vi "布线趋势图示-单根.vi"(0 "基本信息":T2, 1 "布线前甩线":string[][](table), 2 "布线点位":string[][](table), 3 "布线后甩线":string[][](table), 4 "轨迹选择":u16(ring) items=["显示单根轨迹", "显示全部轨迹"]) -> (14 "引用句柄输出":T1)   [LabVIEW 2014]
uses:
  <vilib>/vision/Image Controls.llb/IMAQ Image.ctl
panel:
  out "x-y 2":dbl
  out "x-y":dbl
  out "YMIN":dbl
  out "XMIN":dbl
  out "YMAX":dbl
  out "XMAX":dbl
  out "Image":T1(plugin-control)
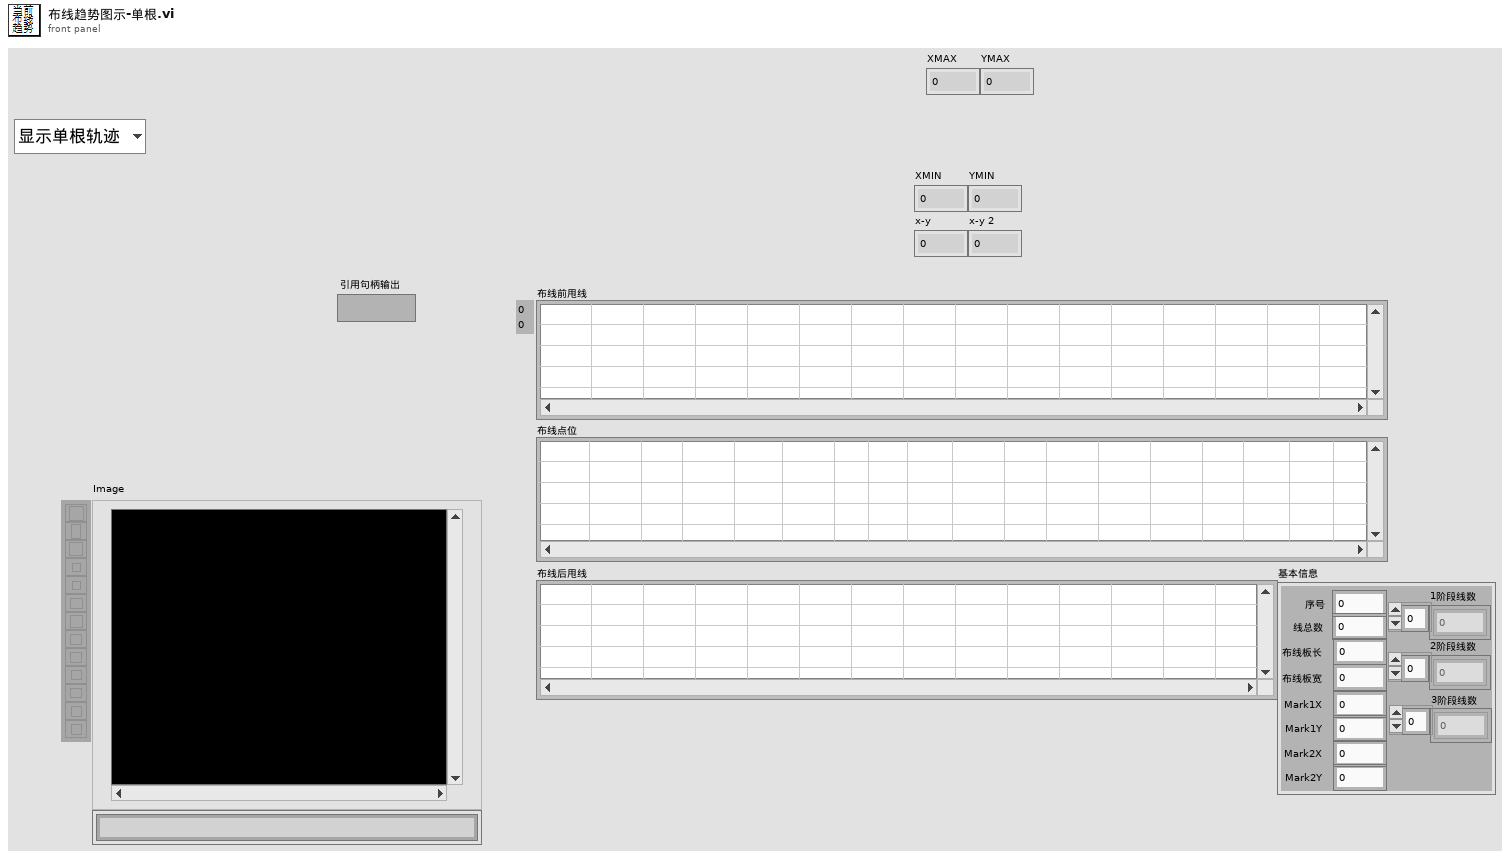
[diagram p1: front panel]
types:
  T1 = typedef "IMAQ Image.ctl" = refnum<image>
  T2 = typedef "基本信息.ctl" = cluster{"序号":dbl, "线总数":dbl, "布线板长":dbl, "布线板宽":dbl, "Mark1X":dbl, "Mark1Y":dbl, "Mark2X":dbl, "Mark2Y":dbl, "1阶段线数":dbl[], "2阶段线数":dbl[], "3阶段线数":dbl[]}
  T3 = typedef "Image Type" = u32
  T4 = cluster{i32, i32, "X Resolution":i32, "Y Resolution":i32}
  T5 = cluster{cluster{"X":dbl, "Y":dbl}, cluster{"X":dbl, "Y":dbl}}
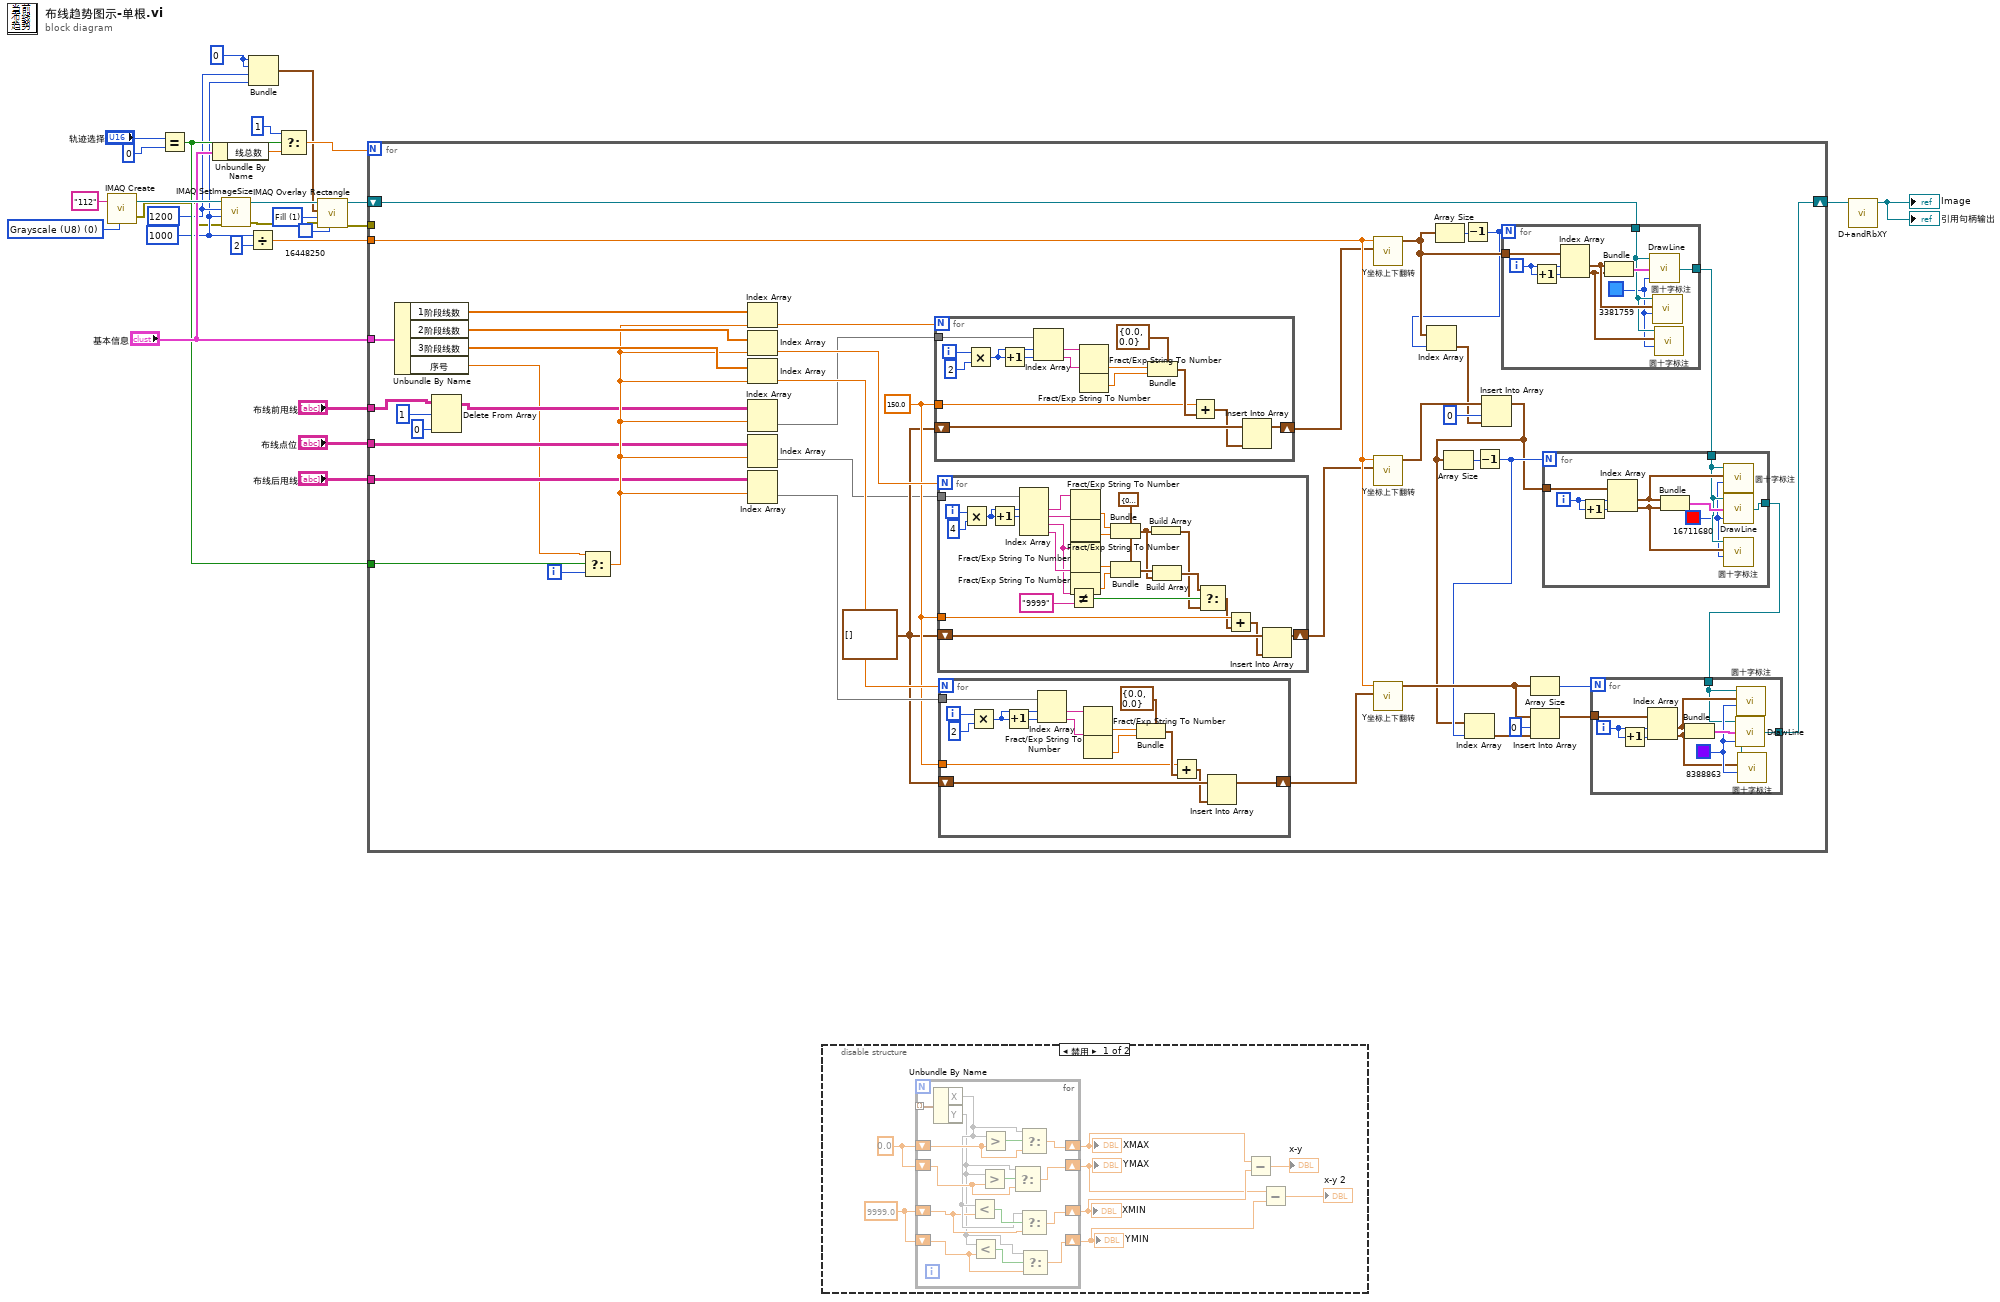
[diagram p0: block diagram]
diagram:
  w8 = 0
  w13 = u32 1 items=["Frame", "Fill", "Highlight"] ("Drawing Mode (Frame)")
  w5 = 1000 ("Y Resolution")
  w6 = 1200 ("X Resolution")
  w27 = T3 0 items=["Grayscale (U8)", "Grayscale (I16)", "Grayscale (SGL)", "Complex (CSG)", "RGB (U32)", "HSL (U32)", "RGB (U64)", "Grayscale (U16)"] ("Image Type")
  n1 = call "IMAQ Create"("Image Name"="112", "Image Type"=w27) -> ("New Image"=w28:T1, "error out"=w3:errorcluster)  [unwired: 3 in]
  n2 = Equal?(x="轨迹选择", y=u16 0) -> (x = y?=w15:bool)
  n3 = Unbundle By Name("基本信息") -> ("线总数"=w16:dbl)
  n4 = call "IMAQ SetImageSize"("error in (no error)"=w3, "Y Resolution"=w5, "X Resolution"=w6, "Image"=w28) -> ("error out"=w4:errorcluster, "Image Out"=w12:T1)  [unwired: 1 in]
  n5 = Divide(x=w5, y=2) -> (x/y=w20:dbl)
  n6 = Bundle(w8, w8, "X Resolution"=w6, "Y Resolution"=w5) -> (w7:T4)  [unwired: 1 in]
  n7 = Select(t=1, s=w15, f=w16) -> (s? t:f=w9:dbl)
  n8 = call "IMAQ Overlay Rectangle"("Color"=u32 16448250, "error in (no error)"=w4, "Drawing Mode (Frame)"=w13, "Rectangle"=w7, "Image"=w12) -> ("error out"=w2:errorcluster, "Image Out"=w11:T1)  [unwired: 5 in]
  n9 = for {
    N: w9 -> [_]
    tunnel: "布线前甩线" -> [w35]
    tunnel: "布线点位" -> [w36]
    tunnel: "布线后甩线" -> [w38]
    tunnel: "基本信息" -> [w72]
    tunnel: w20 -> [w54]
    shift-right: [w56] -> w14
    shift-left: w11 -> [w52]
    tunnel: w15 -> [w47]
    tunnel: w2 -> [_]
    i -> [w45]
    w63 = cluster{"X":dbl, "Y":dbl}[] []
    w64 = 150.0 ("x")
    n10 = Unbundle By Name(w72) -> ("1阶段线数"=w71:dbl[], "2阶段线数"=w70:dbl[], "3阶段线数"=w69:dbl[], "序号"=w29:dbl)
    n11 = Delete From Array(array=w35, length=1 ("长度"), index (col)=0 ("禁用的索引 (列)")) -> (array with subset deleted=w33:string[][])  [unwired: 1 in, 1 out]
    n12 = Select(t=w29, s=w47, f=w45) -> (s? t:f=w46:dbl)
    n13 = Index Array(array=w71, index=w46) -> (element=w67:dbl)
    n14 = Index Array(array=w70, index=w46) -> (element=w66:dbl)
    n15 = Index Array(array=w69, index=w46) -> (element=w65:dbl)
    n16 = Index Array(array=w33, index (row)=w46) -> (element=w32:string[])  [unwired: 1 in]
    n17 = Index Array(array=w36, index (row)=w46) -> (element=w31:string[])  [unwired: 1 in]
    n18 = Index Array(array=w38, index (row)=w46) -> (element=w68:string[])  [unwired: 1 in]
    n19 = for {
      N: w67 -> [_]
      tunnel: w32 -> [w154]
      tunnel: w64 -> [w143]
      shift-right: [w140] -> w50
      shift-left: w63 -> [w142]
      i -> [w153]
      n20 = Multiply(x=w153, y=2) -> (x*y=w151:i32)
      n21 = Increment(x=w151) -> (x+1=w150:i32)
      n22 = Index Array(array=w154, index #1=w151, index #2=w150) -> (element #1=w149:string, element #2=w148:string)
      n23 = Fract/Exp String To Number(string=w149) -> (number=w147:dbl)  [unwired: 3 in, 1 out]
      n24 = Fract/Exp String To Number(string=w148) -> (number=w146:dbl)  [unwired: 3 in, 1 out]
      n25 = Bundle(cluster=cluster{"X":dbl, "Y":dbl} {"X"=0.0, "Y"=0.0}, "X"=w147, "Y"=w146) -> (w144:cluster{"X":dbl, "Y":dbl})
      n26 = Add(x=w143, y=w144) -> (x+y=w141:cluster{"X":dbl, "Y":dbl})
      n27 = Insert Into Array(array=w142, new element=w141) -> (w140:cluster{"X":dbl, "Y":dbl}[])  [unwired: 1 in]
    }
    n28 = for {
      N: w66 -> [_]
      tunnel: w31 -> [w139]
      tunnel: w64 -> [w130]
      shift-right: [w119] -> w48
      shift-left: w63 -> [w120]
      i -> [w138]
      w123 = cluster{"X":dbl, "Y":dbl} {"X"=0.0, "Y"=0.0}
      n29 = Multiply(x=w138, y=4) -> (x*y=w136:i32)
      n30 = Increment(x=w136) -> (x+1=w135:i32)
      n31 = Index Array(array=w139, index #1=w136, index #2=w135) -> (element #1=w134:string, element #2=w133:string, element #3=w115:string, element #4=w128:string)  [unwired: 2 in]
      n32 = Not Equal?(x=w115, y="9999") -> (x != y?=w125:bool)
      n33 = Fract/Exp String To Number(string=w134) -> (number=w132:dbl)  [unwired: 3 in, 1 out]
      n34 = Fract/Exp String To Number(string=w133) -> (number=w131:dbl)  [unwired: 3 in, 1 out]
      n35 = Fract/Exp String To Number(string=w115) -> (number=w127:dbl)  [unwired: 3 in, 1 out]
      n36 = Fract/Exp String To Number(string=w128) -> (number=w126:dbl)  [unwired: 3 in, 1 out]
      n37 = Bundle(cluster=w123, "X"=w132, "Y"=w131) -> (w116:cluster{"X":dbl, "Y":dbl})
      n38 = Bundle(cluster=w123, "X"=w127, "Y"=w126) -> (w117:cluster{"X":dbl, "Y":dbl})
      n39 = Build Array(w116) -> (w122:cluster{"X":dbl, "Y":dbl}[])
      n40 = Build Array(w117, w116) -> (w124:cluster{"X":dbl, "Y":dbl}[])
      n41 = Select(t=w124, s=w125, f=w122) -> (s? t:f=w121:cluster{"X":dbl, "Y":dbl}[])
      n42 = Add(x=w130, y=w121) -> (x+y=w118:cluster{"X":dbl, "Y":dbl}[])
      n43 = Insert Into Array(array=w120, new element=w118) -> (w119:cluster{"X":dbl, "Y":dbl}[])  [unwired: 1 in]
    }
    n44 = for {
      N: w65 -> [_]
      tunnel: w68 -> [w114]
      tunnel: w64 -> [w103]
      shift-right: [w101] -> w49
      shift-left: w63 -> [w102]
      i -> [w113]
      n45 = Multiply(x=w113, y=2) -> (x*y=w111:i32)
      n46 = Increment(x=w111) -> (x+1=w110:i32)
      n47 = Index Array(array=w114, index #1=w111, index #2=w110) -> (element #1=w109:string, element #2=w108:string)
      n48 = Fract/Exp String To Number(string=w109) -> (number=w107:dbl)  [unwired: 3 in, 1 out]
      n49 = Fract/Exp String To Number(string=w108) -> (number=w106:dbl)  [unwired: 3 in, 1 out]
      n50 = Bundle(cluster=cluster{"X":dbl, "Y":dbl} {"X"=0.0, "Y"=0.0}, "X"=w107, "Y"=w106) -> (w104:cluster{"X":dbl, "Y":dbl})
      n51 = Add(x=w103, y=w104) -> (x+y=w100:cluster{"X":dbl, "Y":dbl})
      n52 = Insert Into Array(array=w102, new element=w100) -> (w101:cluster{"X":dbl, "Y":dbl}[])  [unwired: 1 in]
    }
    n53 = call "Y坐标上下翻转.vi"("数组输入"=w50, "数值"=w54) -> ("数组输出"=w44:cluster{"X":dbl, "Y":dbl}[])  [unwired: 9 in]
    n54 = call "Y坐标上下翻转.vi"("数组输入"=w48, "数值"=w54) -> ("数组输出"=w42:cluster{"X":dbl, "Y":dbl}[])  [unwired: 9 in]
    n55 = call "Y坐标上下翻转.vi"("数组输入"=w49, "数值"=w54) -> ("数组输出"=w55:cluster{"X":dbl, "Y":dbl}[])  [unwired: 9 in]
    n56 = Array Size(array=w44) -> (size(s)=w53:i32)
    n57 = Decrement(x=w53) -> (x-1=w43:i32)
    n58 = Index Array(array=w44, index=w43) -> (element=w30:cluster{"X":dbl, "Y":dbl})
    n59 = Insert Into Array(array=w42, index=0 ("索引"), new element=w30) -> (w39:cluster{"X":dbl, "Y":dbl}[])
    n60 = Array Size(array=w39) -> (size(s)=w61:i32)
    n61 = Decrement(x=w61) -> (x-1=w40:i32)
    n62 = Index Array(array=w39, index=w40) -> (element=w60:cluster{"X":dbl, "Y":dbl})
    n63 = for {
      N: w43 -> [_]
      tunnel: w44 -> [w90]
      tunnel: w52 -> [w83]
      tunnel: [w88] -> w51
      i -> [w85]
      w82 = u32 3381759 ("Color")
      n64 = Increment(x=w85) -> (x+1=w86:i32)
      n65 = Index Array(array=w90, index #1=w85, index #2=w86) -> (element #1=w87:cluster{"X":dbl, "Y":dbl}, element #2=w84:cluster{"X":dbl, "Y":dbl})
      n66 = Bundle(w87, w84) -> (w89:T5)  [unwired: 1 in]
      n67 = call "DrawLine.vi"("Color"=w82, "Edge Points"=w89, "img in"=w83) -> ("Image Out"=w88:T1)
      n68 = call "圆十字标注.vi"("Color"=w82, "簇"=w87, "引用句柄输入"=w83) -> ()  [unwired: 8 in, 1 out]
      n69 = call "圆十字标注.vi"("Color"=w82, "簇"=w84, "引用句柄输入"=w83) -> ()  [unwired: 8 in, 1 out]
    }
    n70 = Array Size(array=w55) -> (size(s)=w58:i32)
    n71 = Insert Into Array(array=w55, index=0 ("索引"), new element=w60) -> (w59:cluster{"X":dbl, "Y":dbl}[])
    n72 = for {
      N: w40 -> [_]
      tunnel: w39 -> [w99]
      tunnel: w51 -> [w93]
      tunnel: [w94] -> w62
      i -> [w97]
      w91 = u32 16711680 ("Color")
      n73 = Increment(x=w97) -> (x+1=w96:i32)
      n74 = Index Array(array=w99, index #1=w97, index #2=w96) -> (element #1=w95:cluster{"X":dbl, "Y":dbl}, element #2=w92:cluster{"X":dbl, "Y":dbl})
      n75 = Bundle(w95, w92) -> (w98:T5)  [unwired: 1 in]
      n76 = call "圆十字标注.vi"("Color"=w91, "簇"=w95, "引用句柄输入"=w93) -> ()  [unwired: 8 in, 1 out]
      n77 = call "DrawLine.vi"("Color"=w91, "Edge Points"=w98, "img in"=w93) -> ("Image Out"=w94:T1)
      n78 = call "圆十字标注.vi"("Color"=w91, "簇"=w92, "引用句柄输入"=w93) -> ()  [unwired: 8 in, 1 out]
    }
    n79 = for {
      N: w58 -> [_]
      tunnel: w59 -> [w81]
      tunnel: w62 -> [w73]
      tunnel: [w79] -> w56
      i -> [w78]
      w75 = u32 8388863 ("Color")
      n80 = Increment(x=w78) -> (x+1=w77:i32)
      n81 = Index Array(array=w81, index #1=w78, index #2=w77) -> (element #1=w76:cluster{"X":dbl, "Y":dbl}, element #2=w74:cluster{"X":dbl, "Y":dbl})
      n82 = Bundle(w76, w74) -> (w80:T5)  [unwired: 1 in]
      n83 = call "DrawLine.vi"("Color"=w75, "Edge Points"=w80, "img in"=w73) -> ("Image Out"=w79:T1)
      n84 = call "圆十字标注.vi"("Color"=w75, "簇"=w76, "引用句柄输入"=w73) -> ()  [unwired: 8 in, 1 out]
      n85 = call "圆十字标注.vi"("Color"=w75, "簇"=w74, "引用句柄输入"=w73) -> ()  [unwired: 8 in, 1 out]
    }
  }
  n86 = disable-structure shown="禁用" {
    frame Disabled {
      w161 = 9999.0
      w162 = 0.0
      n87 = for {
        tunnel: _ -> [w177] mode=indexing
        shift-right: [w174] -> w160
        shift-left: w162 -> [w175]
        shift-right: [w171] -> w158
        shift-left: w162 -> [w172]
        shift-right: [w167] -> w159
        shift-left: w161 -> [w168]
        shift-right: [w163] -> w157
        shift-left: w161 -> [w164]
        n88 = Unbundle By Name(w177) -> ("X"=w169, "Y"=w165)
        n89 = Less?(x=w169, y=w168) -> (x < y?=w170:bool)
        n90 = Less?(x=w165, y=w164) -> (x < y?=w166:bool)
        n91 = Greater?(x=w165, y=w172) -> (0:w173:bool)
        n92 = Greater?(x=w169, y=w175) -> (0:w176:bool)
        n93 = Select(t=w165, s=w173, f=w172) -> (s? t:f=w171:dbl)
        n94 = Select(t=w169, s=w176, f=w175) -> (s? t:f=w174:dbl)
        n95 = Select(t=w169, s=w170, f=w168) -> (s? t:f=w167:dbl)
        n96 = Select(t=w165, s=w166, f=w164) -> (s? t:f=w163:dbl)
      }
      "XMAX" <- w160
      "YMAX" <- w158
      "XMIN" <- w159
      "YMIN" <- w157
      n97 = Subtract(x=w160, y=w159) -> (x-y=→"x-y":dbl)
      n98 = Subtract(x=w158, y=w157) -> (x-y=→"x-y 2":dbl)
    }
    frame Enabled {
    }
  }
  n99 = call "D+andRbXY.vi"("引用句柄输入"=w14) -> ("Image Out"=→"引用句柄输出" →"Image":T1)  [unwired: 10 in]
